vi "Initialize_Core.vi"(9 "result":bool, 10 "time/date":timestamp=timestamp(3230114789.968 s since 1904-01-01), 11 "Test Results \nParent Class in":refnum<class "Test Results Base Class.lvclass">) -> (3 "Test Results\nParent Class out":refnum<class "Test Results Base Class.lvclass">)   [LabVIEW 2020, in "Test Results Base Class.lvclass"]
doc: "This VI initializes the data members of the class \"Test Results Parent Class.\" This VI is an example of a protected member VI of a LabVIEW class. Only VIs within the same class or a descendant class can call this VI."
uses:
  Test Results Base Class.lvclass
  Test Results Base Class.lvclass/Test Results Base Class.ctl
panel:
  # "This VI is an example of a protected member VI of a LabVIEW class. Only VIs within\nthe same class or a descendant class can call this VI."
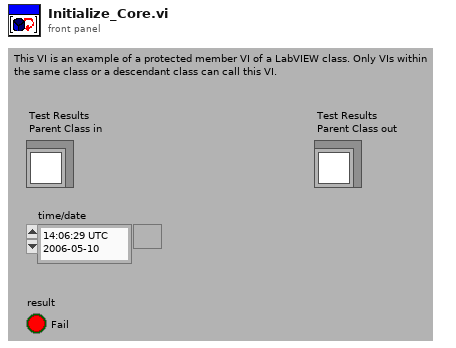
[diagram p1: front panel]
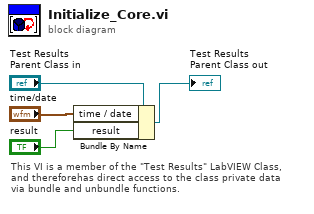
[diagram p0: block diagram]
diagram:
  # "This VI is a member of the \"Test Results\" LabVIEW Class, \nand thereforehas direct access to the class private data\nvia bundle and unbundle functions."
  n1 = Bundle By Name(cluster="Test Results \nParent Class in", "time / date"="time/date", "result"="result") -> (→"Test Results\nParent Class out":refnum<class "Test Results Base Class.lvclass">)
